vi "destroy.vi"(8 "error in (no error)":errorcluster, 11 "console.provider in":refnum<class "console.provider.lvclass">) -> (0 "error out":errorcluster)   [LabVIEW 2021, in "console.provider.lvclass"]
uses:
  console.provider.lvclass
  console.provider.lvclass/console.provider.ctl
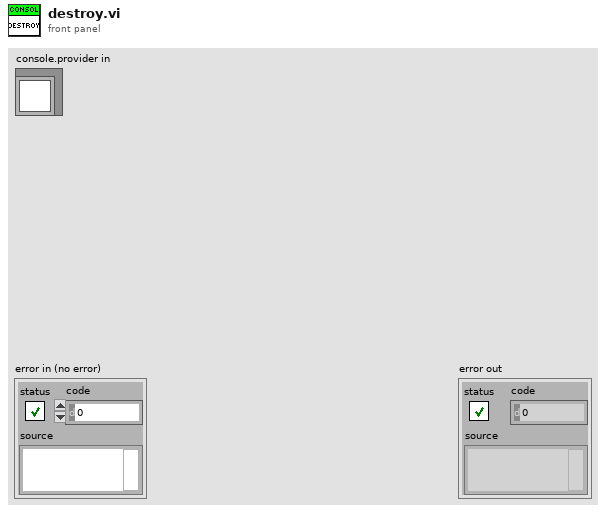
[diagram p1: front panel]
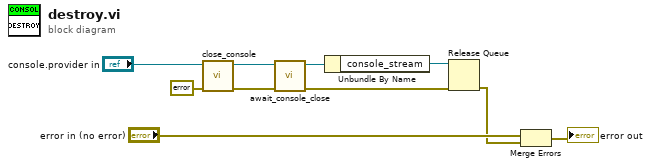
[diagram p0: block diagram]
diagram:
  n1 = call "close_console.vi"("error in (no error)"=errorcluster {"status"=FALSE, "code"=0, "source"=""}, "console.provider in"="console.provider in") -> ("error out"=w6:errorcluster, "console.provider out"=w5:refnum<class "console.provider.lvclass">)  [unwired: 8 in]
  n2 = call "await_console_close.vi"("error in (no error)"=w6, "console.provider in"=w5) -> ("error out"=w2:errorcluster, "console.provider out"=w4:refnum<class "console.provider.lvclass">)  [unwired: 8 in]
  n3 = Unbundle By Name(w4) -> ("console_stream"=w3:refnum<queue>)
  n4 = Release Queue(queue=w3, error in (no error)=w2) -> (error out=w1:errorcluster)  [unwired: 1 in, 2 out]
  n5 = Merge Errors("error in (no error)", w1) -> (→"error out":errorcluster)
